vi "Configure Sample Clock [SC] Core.vi"(8 "error in (no error)":errorcluster, 9 "Sample Clock Source (Internal)":i32(ring) items=["Internal", "External"], 11 "CS++Fgen in":refnum<class "CS++Fgen.lvclass">) -> (0 "error out":errorcluster, 3 "CS++Fgen out":refnum<class "CS++Fgen.lvclass">)   [LabVIEW 2016, in "CS++Fgen.lvlib" / "CS++Fgen.lvclass"]
doc: "This VI configures the sample clock source for the function generator. \n\nNote:\n\n(1) This VI is part of the IviFgenSampleClock [SC] extension group."
uses:
  CS++Fgen.lvclass
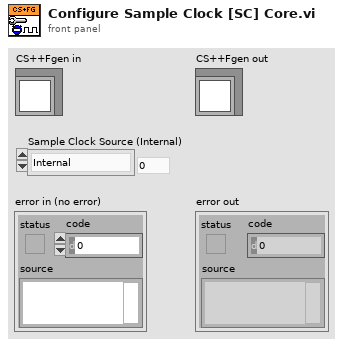
[diagram p1: front panel]
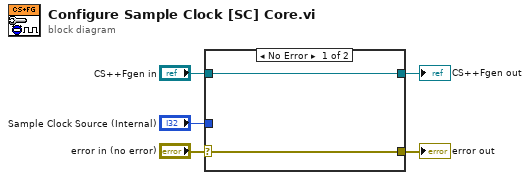
[diagram p0: block diagram]
diagram:
  n1 = case shown="No Error" "error in (no error)" {
    selector: "error in (no error)" -> [w6 w9]
    tunnel: [w6 w9] -> w4
    tunnel: [w7 w8] -> w2
    tunnel: "CS++Fgen in" -> [w7 w8]
    tunnel: "Sample Clock Source (Internal)" -> [_ _]
    frame No Error {
    }
    frame Error {
    }
  }
  "error out" <- w4
  "CS++Fgen out" <- w2
